vi "readAnAlogSettings.vi"(8 "error in (no error)":errorcluster, 10 "output cluster in":T1={"DC Restore"=enum."off", "Polarity"=enum."Negative", "TV Event"=enum."Field 1", "Coupling"=enum."AC", "Slope"=enum."Negative", "AnalogSource"=enum."Channel 0", "Window Mode"=enum."Entering", "Low Level"=0.0, "High Level"=0.0, "Hysteresis"=0.0, "Delay"=0.0, "Holdoff"=0.0, "Signal Format"=enum."M-NTSC", "Mode"=enum."Immediate", "Line Number"=0, "DigitalSource"=enum."RTSI 0"}, 11 "IVI Refnum in":refnum<k15>) -> (0 "error out":errorcluster, 2 "output cluster out":T1={"DC Restore"=enum."off", "Polarity"=enum."Negative", "TV Event"=enum."Field 1", "Coupling"=enum."AC", "Slope"=enum."Negative", "AnalogSource"=enum."Channel 0", "Window Mode"=enum."Entering", "Low Level"=0.0, "High Level"=0.0, "Hysteresis"=0.0, "Delay"=0.0, "Holdoff"=0.0, "Signal Format"=enum."M-NTSC", "Mode"=enum."Immediate", "Line Number"=0, "DigitalSource"=enum."RTSI 0"}, 3 "IVI Refnum out":refnum<k15>)   [LabVIEW 2011]
uses:
  TriggerSettings_TypDef.ctl
  OnOffTypeDef.ctl
  Polarity_TypDEf.ctl
  TVEvent_TypDef.ctl
  coupling_TypDef.ctl
  positive_negatice2_typDef.ctl
  TriggerSource_TypDef.ctl
  triggerwindowmode2_TypDef.ctl
  SignalFormat_TypDef.ctl
  mode_TypDef.ctl
  Trigger.DigitalSource_TypDEf.ctl
panel:
  out "Triggering:Trigger Source":string
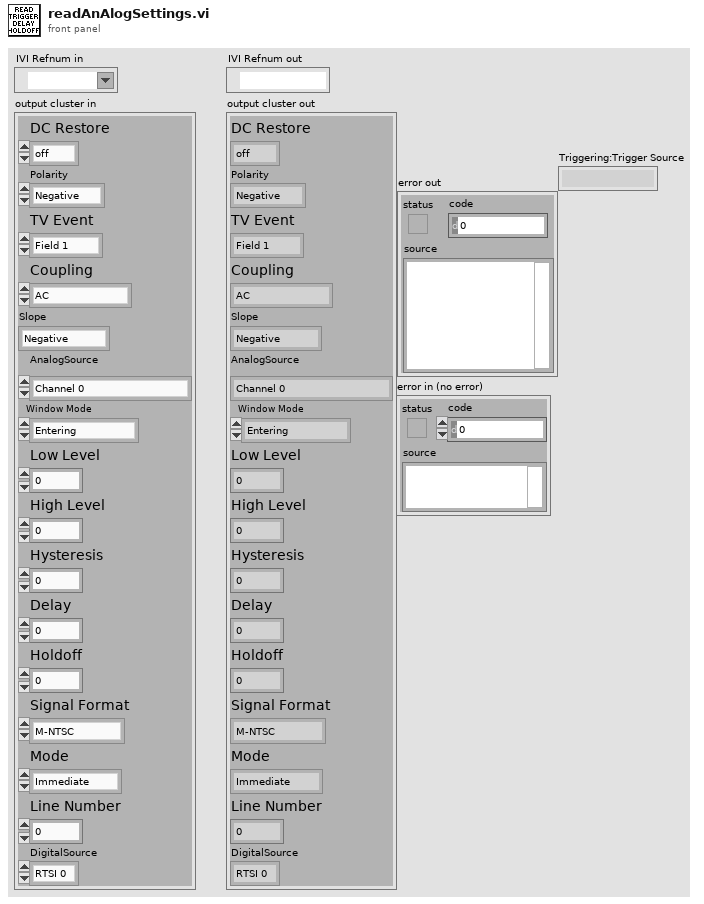
[diagram p1: front panel]
types:
  T1 = typedef "TriggerSettings_TypDef.ctl" = cluster{"DC Restore":T2, "Polarity":T3, "TV Event":T4, "Coupling":T5, "Slope":T6, "AnalogSource":T7, "Window Mode":T8, "Low Level":dbl, "High Level":dbl, "Hysteresis":dbl, "Delay":dbl, "Holdoff":dbl, "Signal Format":T9, "Mode":T10, "Line Number":i32, "DigitalSource":T11}
  T2 = typedef "OnOffTypeDef.ctl" = enum16{"off", "on"}
  T3 = typedef "Polarity_TypDEf.ctl" = enum16{"Negative", "Positive"}
  T4 = typedef "TVEvent_TypDef.ctl" = enum16{"Field 1", "Field 2", "Any Field", "Any Line", "Line Number"}
  T5 = typedef "coupling_TypDef.ctl" = enum16{"AC", "DC", "HF Reject", "LF Reject", "AC Plus HF Reject"}
  T6 = typedef "positive_negatice2_typDef.ctl" = enum16{"Positive", "Negative"}
  T7 = typedef "TriggerSource_TypDef.ctl" = enum16{"Channel 0", "Channel 1", "External TRIG"}
  T8 = typedef "triggerwindowmode2_TypDef.ctl" = enum16{"Entering", "Leaving"}
  T9 = typedef "SignalFormat_TypDef.ctl" = enum16{"M-NTSC", "B/G-PAL", "SECAM", "M-PAL", "480i/59.94 fps", "480i/60 fps", "480p/59.94 Fps", "480p/60 Fps", "576i/50 fps", "576p/50 Fps", "720p/50 Fps", "720p/59.94 Fps", "720p/60 Fps", "1080i/50 fps", "1080i/59.94 fps", "1080i/60 fps", "1080p/24 Fps"}
  T10 = typedef "mode_TypDef.ctl" = enum32{"Immediate", "Analog Edge", "Analog Window", "Analog Hysteresis", "Video", "Digital Edge"}
  T11 = typedef "Trigger.DigitalSource_TypDEf.ctl" = enum16{"RTSI 0", "RTSI 1", "RTSI 2", "RTSI 3", "RTSI 4", "RTSI 5", "RTSI 6", "PFI 0", "PFI 1", "PFI 2", "PXI Star Trigger"}
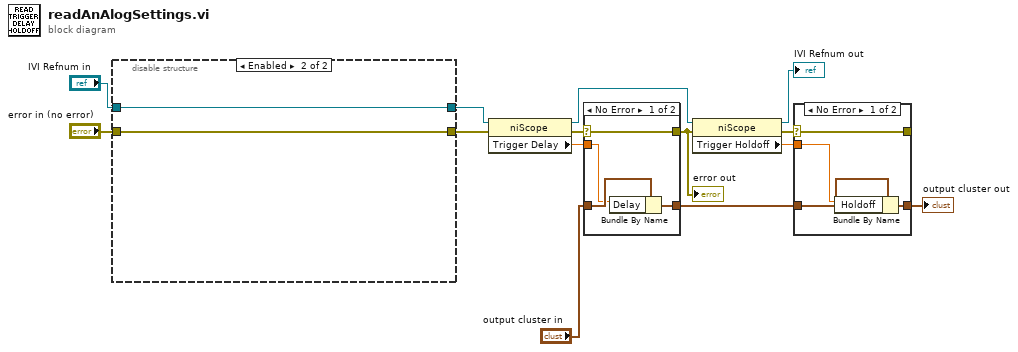
[diagram p0: block diagram]
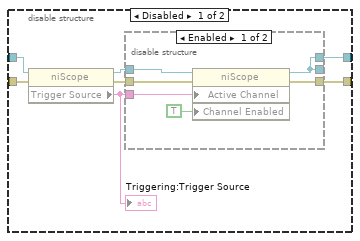
[diagram p3: hidden frame]
diagram:
  n1 = disable-structure shown="Enabled" {
    disable-tunnel: "IVI Refnum in" -> [w18 w31]
    disable-tunnel: [w17 w31] -> w10
    disable-tunnel: "error in (no error)" -> [w16 w30]
    disable-tunnel: [w15 w30] -> w8
    frame Disabled {
      n2 = property class="niScope"(reference=w18, error in=w16) -> (reference out=w21:refnum<k15>, error out=w19:errorcluster, "Trigger Source"=w20:string)
      "Triggering:Trigger Source" <- w20
      n3 = disable-structure shown="Enabled" {
        disable-tunnel: w21 -> [w27 w29]
        disable-tunnel: [w22 w29] -> _
        disable-tunnel: w20 -> [w26 _]
        disable-tunnel: [w25 w28] -> w15
        disable-tunnel: w19 -> [w24 w28]
        disable-tunnel: [w22 _] -> w17
        frame Enabled {
          n4 = property class="niScope"(reference=w27, error in=w24, "Active Channel"=w26, "Channel Enabled"=TRUE ("Vertical:Channel Enabled")) -> (reference out=w22:refnum<k15>, error out=w25:errorcluster)
        }
        frame Disabled {
        }
      }
    }
    frame Enabled {
    }
  }
  n5 = property class="niScope"(reference=w10, error in=w8) -> (reference out=w7:refnum<k15>, error out=w13:errorcluster, "Trigger Delay"=w12:dbl)
  n6 = case shown="No Error" w13 {
    selector: w13 -> [w32 w36]
    tunnel: [w35 w37] -> w2
    tunnel: "output cluster in" -> [w34 w37]
    tunnel: w12 -> [w33 _]
    tunnel: [w32 w36] -> w4
    frame No Error {
      n7 = Bundle By Name(cluster=w34, "Delay"=w33) -> (w35:T1)
    }
    frame Error {
    }
  }
  "error out" <- w4
  n8 = property class="niScope"(reference=w7, error in=w4) -> (reference out=→"IVI Refnum out":refnum<k15>, error out=w5:errorcluster, "Trigger Holdoff"=w3:dbl)
  n9 = case shown="No Error" w5 {
    selector: w5 -> [w38 w42]
    tunnel: [w41 w43] -> w1
    tunnel: w2 -> [w40 w43]
    tunnel: w3 -> [w39 _]
    tunnel: [w38 w42] -> _
    frame No Error {
      n10 = Bundle By Name(cluster=w40, "Holdoff"=w39) -> (w41:T1)
    }
    frame Error {
    }
  }
  "output cluster out" <- w1
